vi "Draw Tree from XML.vi"(1 "xml structure in":T1, 2 "reference":refnum<vi>) -> ()   [LabVIEW 2011]
uses:
  XML Structure - Cluster.ctl
  XML Tag Type - Enum.ctl
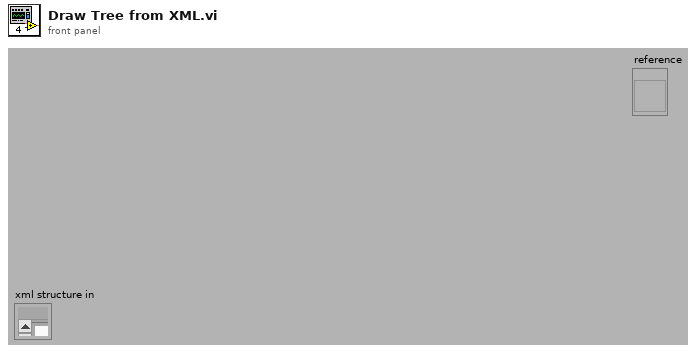
[diagram p1: front panel]
types:
  T1 = typedef "XML Structure - Cluster.ctl" = cluster{"tags":string[], "tag names":string[], "tag type":T2[], "offset":i32[], "close tag index":i32[], "xml":string, "Children":cluster{"children":i32[]}[], "parent index":i32[]}
  T2 = typedef "XML Tag Type - Enum.ctl" = enum16{"start tag", "empty tag", "end tag"}
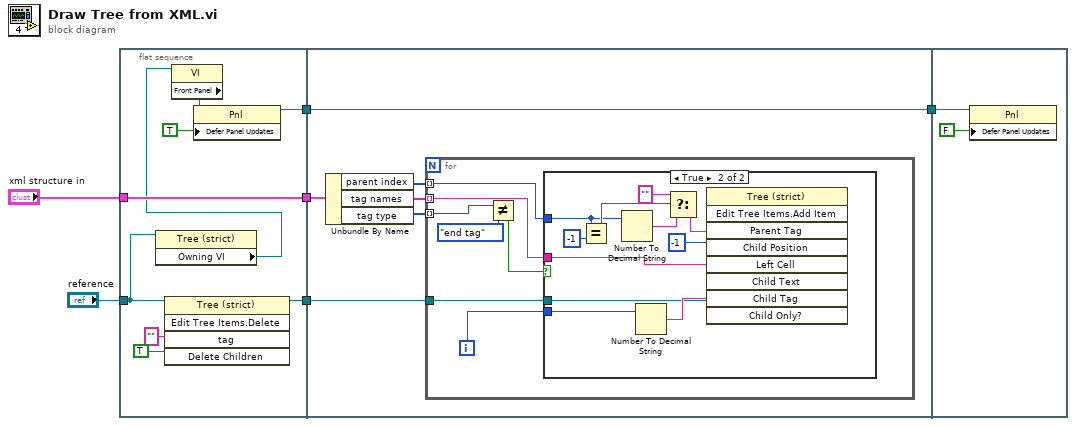
[diagram p0: block diagram]
diagram:
  n1 = flat-sequence {
    tunnel: [w14] -> w6
    tunnel: "reference" -> [w8]
    tunnel: [w10] -> w3
    tunnel: "xml structure in" -> [w10]
    tunnel: [w9] -> w1
    tunnel: [w21] -> w5
    tunnel: w6 -> [w21]
    tunnel: w3 -> [w20]
    tunnel: w1 -> [w16]
    tunnel: w5 -> [w41]
    frame #0 {
      n2 = property class="Tree (strict)"(reference=w8) -> ("Owning VI"=w7:refnum<vi>)  [unwired: 1 in, 2 out]
      n3 = invoke on="Invoke Node" class="Tree (strict)" method="Edit Tree Items.Delete"(reference=w8, "tag"="", "Delete Children"=TRUE) -> (reference out=w9:refnum<vi>)  [unwired: 2 in, 4 out]
      n4 = property class="VI"(reference=w7) -> ("Front Panel"=w15:refnum<vi>)  [unwired: 1 in, 2 out]
      n5 = property class="Pnl"(reference=w15, "Defer Panel Updates"=TRUE) -> (reference out=w14:refnum<vi>)  [unwired: 1 in, 1 out]
    }
    frame #1 {
      n6 = Unbundle By Name(w20) -> ("parent index"=w19:i32[], "tag names"=w18:string[], "tag type"=w17:T2[])
      n7 = for {
        tunnel: w16 -> [w27]
        tunnel: w19 -> [w26] mode=indexing
        tunnel: w18 -> [w25] mode=indexing
        tunnel: w17 -> [w23] mode=indexing
        i -> [w28]
        n8 = Not Equal?(x=w23, y=XML_Tag_Type_-_Enum."end tag") -> (x != y?=w22:bool)
        n9 = case shown="True" w22 {
          tunnel: w28 -> [_ w31]
          tunnel: w25 -> [_ w37]
          tunnel: w26 -> [_ w29]
          tunnel: w27 -> [_ w33]
          frame False {
          }
          frame True {
            n10 = Equal?(x=w29, y=-1) -> (x = y?=w30:bool)
            n11 = Number To Decimal String(number=w29) -> (decimal integer string=w36:string)  [unwired: 1 in]
            n12 = Number To Decimal String(number=w31) -> (decimal integer string=w38:string)  [unwired: 1 in]
            n13 = Select(t="", s=w30, f=w36) -> (s? t:f=w35:string)
            n14 = invoke on="Invoke Node" class="Tree (strict)" method="Edit Tree Items.Add Item"(reference=w33, "Parent Tag"=w35, "Child Position"=-1, "Left Cell"=w37, "Child Tag"=w38) -> ()  [unwired: 4 in, 9 out]
          }
        }
      }
    }
    frame #2 {
      n15 = property class="Pnl"(reference=w41, "Defer Panel Updates"=FALSE) -> ()  [unwired: 1 in, 2 out]
    }
  }
